vi "Create Directory.vi"(8 "Error IN":errorcluster, 11 "Default Save Directory IN":path) -> (0 "Error OUT":errorcluster, 3 "Save Directory OUT":path)   [LabVIEW 2018]
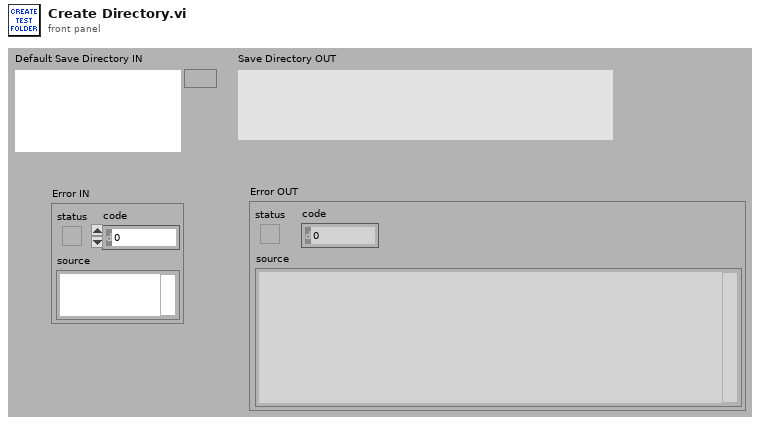
[diagram p1: front panel]
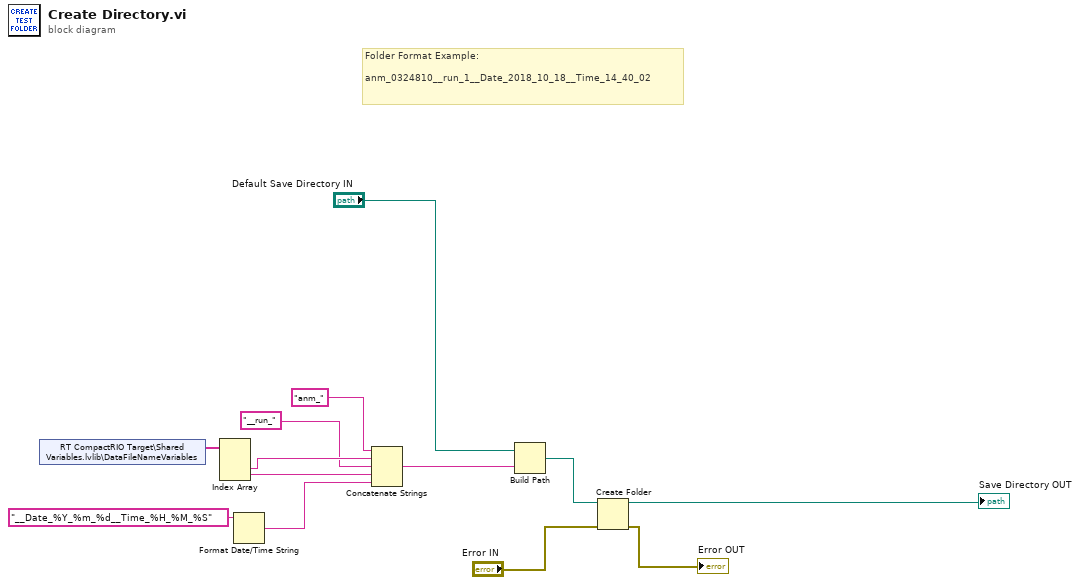
[diagram p0: block diagram]
diagram:
  # "Folder Format Example:\n\nanm_0324810__run_1__Date_2018_10_18__Time_14_40_02"
  n1 = shared-variable "RT CompactRIO Target\\Shared Variables.lvlib\\DataFileNameVariables"() -> (w12:string[])  [unwired: 1 in, 1 out]
  n2 = Index Array(array=w12) -> (element #2=w10:string, element #3=w8:string)  [unwired: 3 in, 1 out]
  n3 = Format Date/Time String(time format string (%c)="__Date_%Y_%m_%d__Time_%H_%M_%S") -> (date/time string=w7:string)  [unwired: 2 in]
  n4 = Concatenate Strings("anm_", w10, "__run_", w8, w7) -> (w5:string)
  n5 = Build Path(base path="Default Save Directory IN", name or relative path=w5) -> (appended path=w4:path)
  n6 = Create Folder(path (use dialog)=w4, error in="Error IN") -> (created path=→"Save Directory OUT":path, error out=→"Error OUT":errorcluster)  [unwired: 2 out]
